vi "ScanType.vi"(8 "error in (no error)":errorcluster, 11 "Type String":string) -> (0 "error out":errorcluster, 3 "SR Type":T1=enum."OPC Servers")   [LabVIEW 2017, in "Client.lvlib" / "ParserSorter.lvlib"]
uses:
  ParserSorter.lvlib
  TypeDefs/SRType.ctl
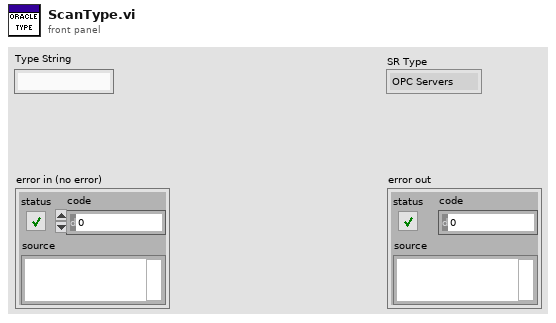
[diagram p1: front panel]
types:
  T1 = typedef "Client.lvlib/ParserSorter.lvlib/SRType.ctl" = enum32{"NaN", "ATE Core Configurations (BYOATE)", "Activation", "BioBench", "CAN", "CM C Series", "Calibration", "Consulting Services", "CounterTimer", "DAQExpress", "DASYLab", "DIAdem", "DMM", "DSA HW", "Digital_IO", "FIRST (NIC Only)", "FieldBus", "FieldPoint", "Functional Savety", "GATI", "GPIB", "HMI and Industrial PCs", "HiQ", "HighSpeedDigital_IO", "IMAQ", "IOTech Vibration", "Industrial Communications", "InsightCM", "LV", "LV CD&Sim", "LV Comms", "LV Controls Add-Ons", "LV Embedded", "LV MathScript RT", "LV NXG", "LV NXT", "LVDSC", "LVFPGA", "LVPDA and LV Touch Panel", "LVRT", "LabWindows_CVI", "Lookout", "MATRIXx", "MStudioDotNet", "MStudioVisualBasic", "MStudioVisualC", "Measure (Legacy)", "Motion", "MultifunctionDAQ", "Multimedia Test HW/SW", "Multisim (EWB)", "NI Update Service", "OPC Servers", "Optical (OSI)", "PXI Controllers, Chassis, MXI", "PXI Timing and Sync", "Power Supplies and SMUs", "Powertrain Controls", "RAID", "RF", "RF Software", "RIO", "SC Express", "SCC", "SCXI", "SPEEDY-33 (Hyperception)", "STS", "ScopeDigitizers", "Serial", "Signal Sources", "SignalCondOther", "SignalExpress", "Software Defined Intruments", "Sound and Vibration SW", "Switch Executive", "Switches", "TestStand", "USRP", "Ultiboard (EWB)", "VBench", "VI Logger", "VXI_MXI", "VeriStand", "VisionSW", "VolumeLicenseMgr", "WSN", "Web UI Builder", "myRIO"}
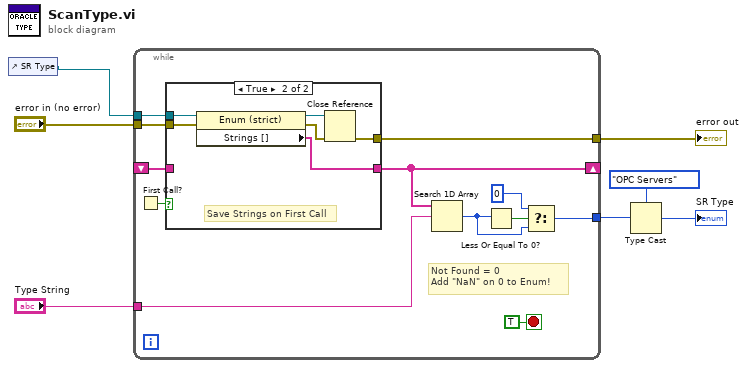
[diagram p0: block diagram]
diagram:
  n1 = control-ref of="SR Type"() -> (w1:refnum<vi>)
  n2 = while {
    tunnel: w1 -> [w19]
    shift-right: [w13] -> _
    shift-left: _ -> [w16]
    tunnel: [w15] -> w6
    tunnel: "error in (no error)" -> [w14]
    tunnel: [w9] -> w4
    tunnel: "Type String" -> [w8]
    stop <- TRUE stop-if-true
    # "Not Found = 0\nAdd \"NaN\" on 0 to Enum!"
    n3 = First Call?() -> (First Call?: T/F=w18:bool)
    n4 = case shown="True" w18 {
      tunnel: w19 -> [_ w27]
      tunnel: [w21 w25] -> w13
      tunnel: w16 -> [w21 _]
      tunnel: [w20 w23] -> w15
      tunnel: w14 -> [w20 w22]
      frame False {
      }
      frame True {
        # "Save Strings on First Call"
        n5 = property class="Enum (strict)"(reference=w27, error in=w22) -> (reference out=w26:refnum<vi>, error out=w24:errorcluster, "Strings []"=w25:string[])
        n6 = Close Reference(reference=w26, error in (no error)=w24) -> (error out=w23:errorcluster)
      }
    }
    n7 = Search 1D Array(1D array=w13, element=w8) -> (index of element=w10:i32)  [unwired: 1 in]
    n8 = Less Or Equal To 0?(x=w10) -> (x <= 0?=w12:bool)
    n9 = Select(t=0 ("Enum Index"), s=w12, f=w10) -> (s? t:f=w9:i32)
  }
  "error out" <- w6
  n10 = Type Cast(type=SRType."OPC Servers" ("SR Type"), x=w4) -> (*(type *) &x=→"SR Type":T1)
